vi "optionalInitialize.vi"(8 "error in (no error)":errorcluster, 10 "Class Name":string, 11 "FPGADMAChannelData in":refnum<class "FPGADMAChannelData.lvclass">) -> (0 "error out":errorcluster, 2 "optional Data":variant, 3 "FPGADMAChannelData out":refnum<class "FPGADMAChannelData.lvclass">)   [LabVIEW 2013, in "FPGADMAChannelData.lvclass"]
uses:
  FPGADMAChannelData.lvclass
  PWM_Specific Data.ctl
  xCE/xceRootNode/xceRootNode.lvclass/xceRootNode.ctl
  xCE/xceRootNode/xceRootNode.lvclass
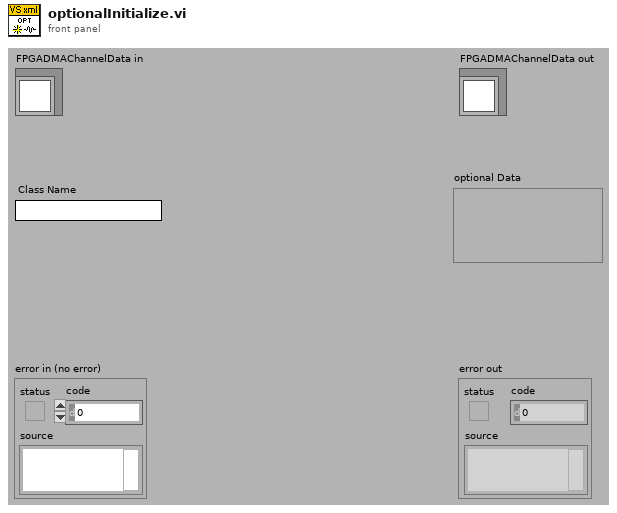
[diagram p1: front panel]
types:
  T1 = typedef "FPGADMAChannelData.lvclass/PWM_Specific Data.ctl" = cluster{"# of parameters":i32, "CnfgEditorDir":path}
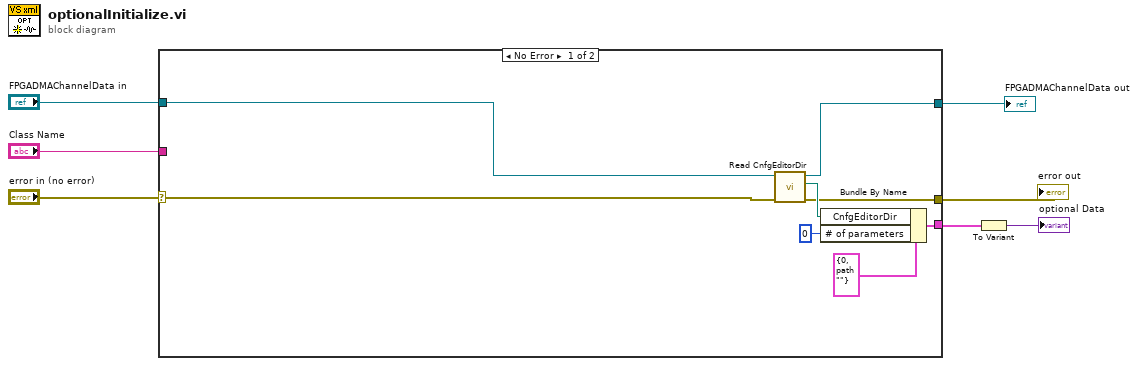
[diagram p0: block diagram]
diagram:
  n1 = case shown="No Error" "error in (no error)" {
    selector: "error in (no error)" -> [w8 w16]
    tunnel: "Class Name" -> [_ _]
    tunnel: "FPGADMAChannelData in" -> [w9 w17]
    tunnel: [w12 w16] -> w1
    tunnel: [w11 _] -> w4
    tunnel: [w14 w17] -> w2
    frame No Error {
      n2 = call "Read CnfgEditorDir.vi"("error in (no error)"=w8, "xceRootNode in"=w9) -> ("error out"=w12:errorcluster, "CnfgEditorDir"=w13:path, "xceRootNode out"=w14:refnum<class "FPGADMAChannelData.lvclass">)  [unwired: 7 in]
      n3 = Bundle By Name(cluster=T1 {"# of parameters"=0, "CnfgEditorDir"=path ""} ("Cluster"), "CnfgEditorDir"=w13, "# of parameters"=0) -> (w11:T1)
    }
    frame Error {
    }
  }
  "error out" <- w1
  "FPGADMAChannelData out" <- w2
  n4 = To Variant(anything=w4) -> (Variant=→"optional Data":variant)
